vi "Save Report Information.vi"(8 "error in (no error)":errorcluster, 10 "Report Information.lvclass":refnum<class "Report Information.lvclass">, 11 "csv-formatter in":refnum<class "csv-formatter.lvclass">) -> (0 "error out":errorcluster, 3 "csv-formatter out":refnum<class "csv-formatter.lvclass">)   [LabVIEW 2015, in "csv-formatter.lvclass"]
doc: "This VI will take the Report Information, format it and write it to the permanent report."
uses:
  csv-formatter.lvclass
  Report Information/Report Information.lvclass
  csv-formatter.lvclass/csv-formatter.ctl
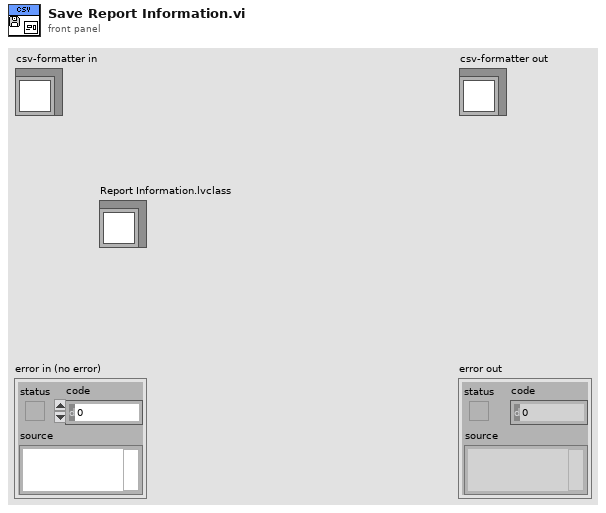
[diagram p1: front panel]
types:
  T1 = typedef "Report Information.lvclass/DUT Information.ctl" = cluster{"DUT Serial Number":string, "DUT Info":string}
  T2 = typedef "Report Information.lvclass/Station Information.ctl" = cluster{"Station ID":string, "Station Serial Number":string}
  T3 = typedef "Report Information.lvclass/Test Information.ctl" = cluster{"UUT Result":string}
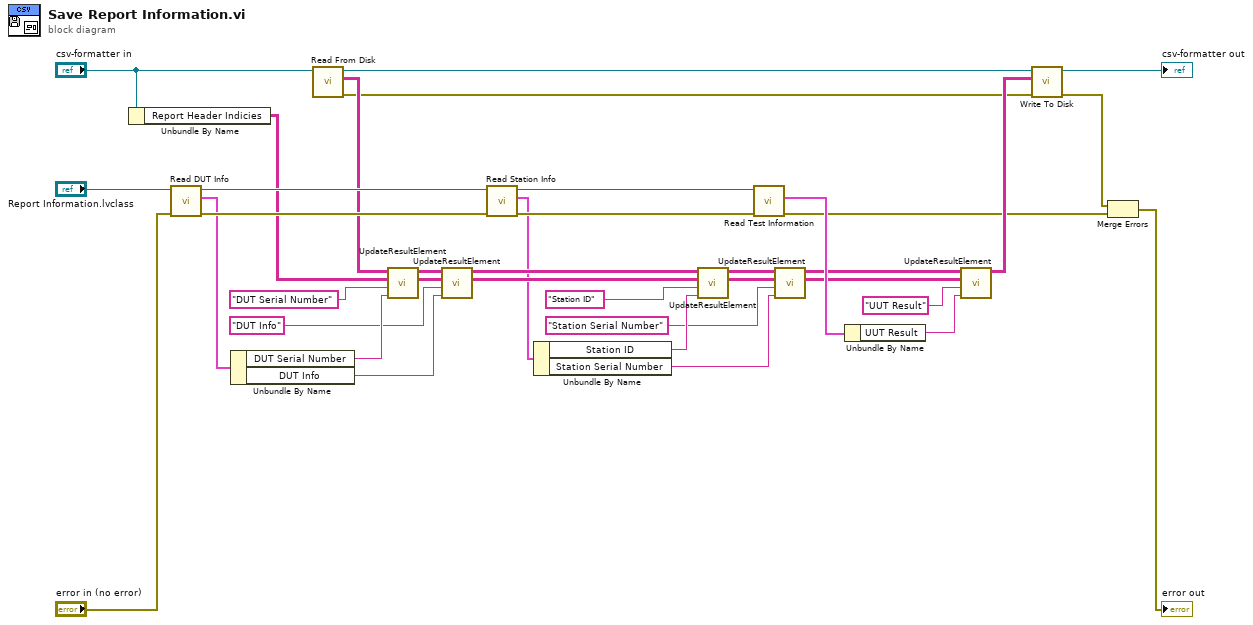
[diagram p0: block diagram]
diagram:
  n1 = Unbundle By Name("csv-formatter in") -> ("Report Header Indicies"=w22:string[][])
  n2 = call-dynamic "Read DUT Info.vi"("error in (no error)"="error in (no error)", "Report Information in"="Report Information.lvclass") -> ("error out"=w32:errorcluster, "DUT Info"=w29:T1, "Report Information out"=w36:refnum<class "Report Information.lvclass">)  [unwired: 7 in]
  n3 = Unbundle By Name(w29) -> ("DUT Serial Number"=w26:string, "DUT Info"=w25:string)
  n4 = call "Read From Disk.vi"("csv-formatter in"="csv-formatter in") -> ("error out"=w1:errorcluster, "Result Out"=w24:string[][], "csv-formatter out"=w31:refnum<class "csv-formatter.lvclass">)  [unwired: 8 in]
  n5 = call "UpdateResultElement.vi"("Data"=w26, "Lookup String"="DUT Serial Number", "Report Header Indicies in"=w22, "Result in"=w24) -> ("Report Header Indicies out"=w21:string[][], "Result Out"=w28:string[][])  [unwired: 6 in]
  n6 = call "UpdateResultElement.vi"("Data"=w25, "Lookup String"="DUT Info", "Report Header Indicies in"=w21, "Result in"=w28) -> ("Report Header Indicies out"=w20:string[][], "Result Out"=w27:string[][])  [unwired: 6 in]
  n7 = call-dynamic "Read Station Info.vi"("error in (no error)"=w32, "Report Information in"=w36) -> ("error out"=w34:errorcluster, "Station Info"=w15:T2, "Report Information out"=w35:refnum<class "Report Information.lvclass">)  [unwired: 7 in]
  n8 = Unbundle By Name(w15) -> ("Station ID"=w14:string, "Station Serial Number"=w13:string)
  n9 = call "UpdateResultElement.vi"("Data"=w14, "Lookup String"="Station ID", "Report Header Indicies in"=w20, "Result in"=w27) -> ("Report Header Indicies out"=w19:string[][], "Result Out"=w18:string[][])  [unwired: 6 in]
  n10 = call-dynamic "Read Test Information.vi"("error in (no error)"=w34, "Report Information in"=w35) -> ("error out"=w4:errorcluster, "Test Information"=w10:T3)  [unwired: 7 in, 1 out]
  n11 = call "UpdateResultElement.vi"("Data"=w13, "Lookup String"="Station Serial Number", "Report Header Indicies in"=w19, "Result in"=w18) -> ("Report Header Indicies out"=w8:string[][], "Result Out"=w9:string[][])  [unwired: 6 in]
  n12 = Unbundle By Name(w10) -> ("UUT Result"=w6:string)
  n13 = call "UpdateResultElement.vi"("Data"=w6, "Lookup String"="UUT Result", "Report Header Indicies in"=w8, "Result in"=w9) -> ("Result Out"=w7:string[][])  [unwired: 6 in, 1 out]
  n14 = call "Write To Disk.vi"("error in (no error)"=w1, "Result In"=w7, "csv-formatter in"=w31) -> ("error out"=w2:errorcluster, "csv-formatter out"=→"csv-formatter out":refnum<class "csv-formatter.lvclass">)  [unwired: 7 in]
  n15 = Merge Errors(w2, w4) -> (→"error out":errorcluster)
